vi "Init ST5520.vi"(8 "error in (no error)":errorcluster caption="entrée d'erreur (pas d'erreur)") -> (0 "error out":errorcluster caption="sortie d'erreur", 3 "Cluster Paramètres fichier Ini":T1)   [LabVIEW 2020]
uses:
  <vilib>/Utility/config.llb/Read Key (U32).vi
  <vilib>/Utility/config.llb/Read Key (String).vi
  <vilib>/Utility/config.llb/Read Key (Double).vi
  <vilib>/Utility/config.llb/NI_LVConfig.lvlib
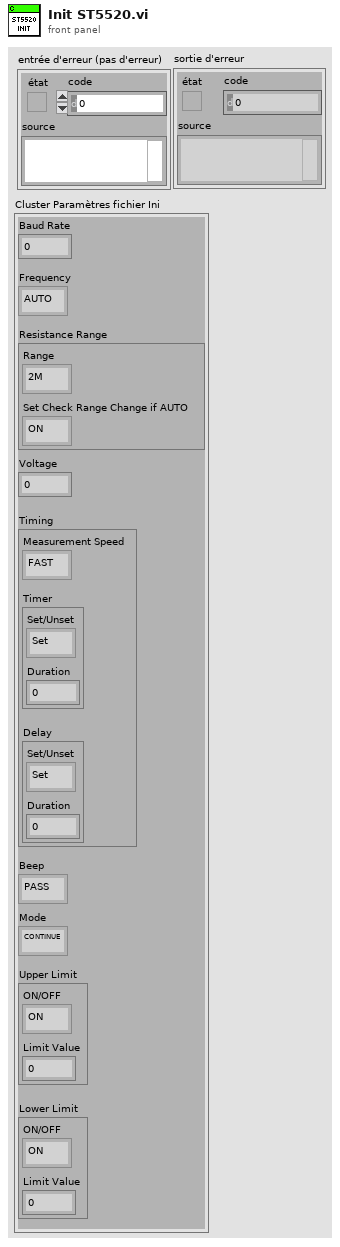
[diagram p1: front panel]
types:
  T1 = cluster{"Baud Rate":u32, "Frequency":enum8{"AUTO", "50", "60"}, "Resistance Range":cluster{"Range":enum16{"2M", "20M", "200M", "2000M", "4000M", "AUTO"}, "Set Check Range Change if AUTO":enum16{"ON", "OFF"}}, "Voltage":u16, "Timing":cluster{"Measurement Speed":enum16{"FAST", "SLOW"}, "Timer":cluster{"Set/Unset":enum8{"Set", "Unset"}, "Duration":dbl}, "Delay":cluster{"Set/Unset":enum8{"Set", "Unset"}, "Duration":dbl}}, "Beep":enum8{"PASS", "FAIL", "OFF", "END"}, "Mode":enum8{"CONTINUE", "PASSSTOP", "FAILSTOP", "SEQUENCE"}, "Upper Limit":cluster{"ON/OFF":enum8{"ON", "OFF"}, "Limit Value":dbl}, "Lower Limit":cluster{"ON/OFF":enum8{"ON", "OFF"}, "Limit Value":dbl}}
  T2 = cluster{"ON/OFF":enum8{"ON", "OFF"}, "Limit Value":dbl}
  T3 = cluster{"Measurement Speed":enum16{"FAST", "SLOW"}, "Timer":cluster{"Set/Unset":enum8{"Set", "Unset"}, "Duration":dbl}, "Delay":cluster{"Set/Unset":enum8{"Set", "Unset"}, "Duration":dbl}}
  T4 = cluster{"Set/Unset":enum8{"Set", "Unset"}, "Duration":dbl}
  T5 = cluster{"Range":enum16{"2M", "20M", "200M", "2000M", "4000M", "AUTO"}, "Set Check Range Change if AUTO":enum16{"ON", "OFF"}}
  T6 = enum8{"CONTINUE", "PASSSTOP", "FAILSTOP", "SEQUENCE"}
  T7 = enum16{"2M", "20M", "200M", "2000M", "4000M", "AUTO"}
  T8 = typedef "NI_LVConfig.lvlib/Config Data RefNum.ctl" = refnum<k1>
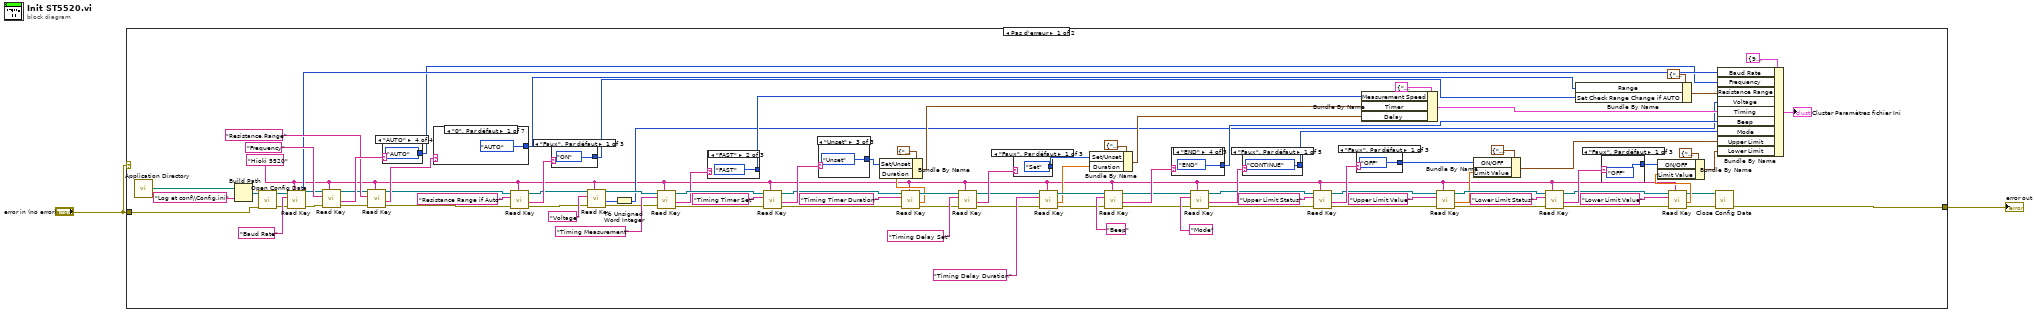
[diagram p0: block diagram]
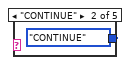
[diagram p2: hidden frame]
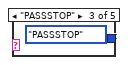
[diagram p3: hidden frame]
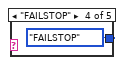
[diagram p4: hidden frame]
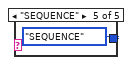
[diagram p5: hidden frame]
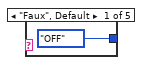
[diagram p6: hidden frame]
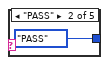
[diagram p7: hidden frame]
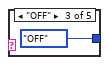
[diagram p8: hidden frame]
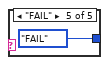
[diagram p9: hidden frame]
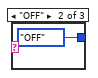
[diagram p10: hidden frame]
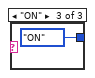
[diagram p11: hidden frame]
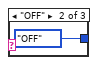
[diagram p12: hidden frame]
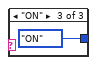
[diagram p13: hidden frame]
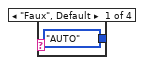
[diagram p14: hidden frame]
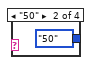
[diagram p15: hidden frame]
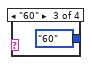
[diagram p16: hidden frame]
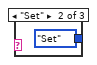
[diagram p17: hidden frame]
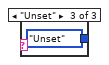
[diagram p18: hidden frame]
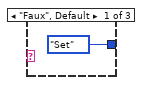
[diagram p19: hidden frame]
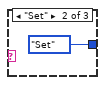
[diagram p20: hidden frame]
diagram:
  n1 = case shown="Pas d'erreur" "error in (no error)" {
    tunnel: "error in (no error)" -> [w5 w139]
    tunnel: [w4 w139] -> w2
    frame No Error {
      w7 = "Hioki 5520" ("section")
      n2 = call <vilib>:"Application Directory.vi"() -> ("Application Directory"=w3:path)
      n3 = Build Path(base path=w3, name or relative path="Log et conf\\Config.ini") -> (appended path=w43:path)
      n4 = call <vilib>:"Open Config Data.vi"("error in (no error)"=w5, "configuration file path"=w43) -> ("error out"=w6:errorcluster, "refnum"=w45:T8)  [unwired: 7 in, 1 out]
      n5 = call-poly <vilib>:"Read Key.vi"("section"=w7, "error in (no error)"=w6, "key"="Baud Rate", "refnum"=w45) -> ("error out"=w16:errorcluster, "value"=w41:u32, "refnum out"=w47:T8)  [unwired: 4 in, 1 out]
      n6 = call-poly <vilib>:"Read Key.vi"("section"=w7, "error in (no error)"=w16, "key"="Frequency", "refnum"=w47) -> ("error out"=w15:errorcluster, "value"=w68:string, "refnum out"=w48:T8)  [unwired: 4 in, 1 out]
      n7 = call-poly <vilib>:"Read Key.vi"("section"=w7, "error in (no error)"=w15, "key"="Resistance Range", "refnum"=w48) -> ("error out"=w14:errorcluster, "value"=w64:string, "refnum out"=w49:T8)  [unwired: 4 in, 1 out]
      n8 = case shown="\"AUTO\"" w68 {
        tunnel: [enum8{"AUTO", "50", "60"}."AUTO" ("Frequency") enum8{"AUTO", "50", "60"}."50" ("Frequency") enum8{"AUTO", "50", "60"}."60" ("Frequency") enum8{"AUTO", "50", "60"}."AUTO" ("Frequency")] -> w40
        frame "Faux", Default {
        }
        frame "50" {
        }
        frame "60" {
        }
        frame "AUTO" {
        }
      }
      n9 = case shown="\"0\", Par défaut" w64 {
        tunnel: [T7."AUTO" ("Range") T7."2M" ("Range") T7."20M" ("Range") T7."200M" ("Range") T7."2000M" ("Range") T7."4000M" ("Range") T7."AUTO" ("Range")] -> w39
        frame "0", Default {
        }
        frame "2M" {
        }
        frame "20M" {
        }
        frame "200M" {
        }
        frame "2000M" {
        }
        frame "4000M" {
        }
        frame "AUTO" {
        }
      }
      n10 = call-poly <vilib>:"Read Key.vi"("section"=w7, "error in (no error)"=w14, "key"="Resistance Range if Auto", "refnum"=w49) -> ("error out"=w13:errorcluster, "value"=w65:string, "refnum out"=w50:T8)  [unwired: 4 in, 1 out]
      n11 = case shown="\"Faux\", Par défaut" w65 {
        tunnel: [enum16{"ON", "OFF"}."ON" ("Set Check Range Change if AUTO") enum16{"ON", "OFF"}."ON" ("Set Check Range Change if AUTO") enum16{"ON", "OFF"}."OFF" ("Set Check Range Change if AUTO")] -> w38
        frame "Faux", Default {
        }
        frame "ON" {
        }
        frame "OFF" {
        }
      }
      n12 = call-poly <vilib>:"Read Key.vi"("section"=w7, "error in (no error)"=w13, "key"="Voltage", "refnum"=w50) -> ("error out"=w12:errorcluster, "value"=w27:u32, "refnum out"=w51:T8)  [unwired: 4 in, 1 out]
      n13 = To Unsigned Word Integer(number=w27) -> (unsigned 16bit integer=w26:u16)
      n14 = call-poly <vilib>:"Read Key.vi"("section"=w7, "error in (no error)"=w12, "key"="Timing Measurement", "refnum"=w51) -> ("error out"=w11:errorcluster, "value"=w46:string, "refnum out"=w52:T8)  [unwired: 4 in, 1 out]
      n15 = case shown="\"FAST\"" w46 {
        tunnel: [enum16{"FAST", "SLOW"}."SLOW" ("Measurement Speed") enum16{"FAST", "SLOW"}."FAST" ("Measurement Speed") enum16{"FAST", "SLOW"}."SLOW" ("Measurement Speed")] -> w37
        frame "Faux", Default {
        }
        frame "FAST" {
        }
        frame "SLOW" {
        }
      }
      n16 = call-poly <vilib>:"Read Key.vi"("section"=w7, "error in (no error)"=w11, "key"="Timing Timer Set", "refnum"=w52) -> ("error out"=w10:errorcluster, "value"=w66:string, "refnum out"=w53:T8)  [unwired: 4 in, 1 out]
      n17 = case shown="\"Unset\"" w66 {
        tunnel: [enum8{"Set", "Unset"}."Set" ("Set/Unset") enum8{"Set", "Unset"}."Set" ("Set/Unset") enum8{"Set", "Unset"}."Unset" ("Set/Unset")] -> w36
        frame "Faux", Default {
        }
        frame "Set" {
        }
        frame "Unset" {
        }
      }
      n18 = call-poly <vilib>:"Read Key.vi"("section"=w7, "error in (no error)"=w10, "key"="Timing Timer Duration", "refnum"=w53) -> ("error out"=w9:errorcluster, "value"=w30:dbl, "refnum out"=w63:T8)  [unwired: 4 in, 1 out]
      n19 = Bundle By Name(cluster=T4 {"Set/Unset"=enum."Set", "Duration"=60.0} ("Timer"), "Set/Unset"=w36, "Duration"=w30) -> (w90:T4)
      n20 = call-poly <vilib>:"Read Key.vi"("section"=w7, "error in (no error)"=w9, "key"="Timing Delay Set", "refnum"=w63) -> ("error out"=w8:errorcluster, "value"=w67:string, "refnum out"=w54:T8)  [unwired: 4 in, 1 out]
      n21 = case shown="\"Faux\", Par défaut" w67 {
        tunnel: [enum8{"Set", "Unset"}."Set" ("Set/Unset") enum8{"Set", "Unset"}."Set" ("Set/Unset") enum8{"Set", "Unset"}."Unset" ("Set/Unset")] -> w86
        frame "Faux", Default {
        }
        frame "Set" {
        }
        frame "Unset" {
        }
      }
      n22 = call-poly <vilib>:"Read Key.vi"("section"=w7, "error in (no error)"=w8, "key"="Timing Delay Duration", "refnum"=w54) -> ("error out"=w17:errorcluster, "value"=w29:dbl, "refnum out"=w69:T8)  [unwired: 4 in, 1 out]
      n23 = Bundle By Name(cluster=T4 {"Set/Unset"=enum."Set", "Duration"=0.0} ("Delay"), "Set/Unset"=w86, "Duration"=w29) -> (w91:T4)
      n24 = call-poly <vilib>:"Read Key.vi"("section"=w7, "error in (no error)"=w17, "key"="Beep", "refnum"=w69) -> ("error out"=w18:errorcluster, "value"=w83:string, "refnum out"=w76:T8)  [unwired: 4 in, 1 out]
      n25 = case shown="\"END\"" w83 {
        tunnel: [enum8{"PASS", "FAIL", "OFF", "END"}."OFF" ("Beep") enum8{"PASS", "FAIL", "OFF", "END"}."PASS" ("Beep") enum8{"PASS", "FAIL", "OFF", "END"}."OFF" ("Beep") enum8{"PASS", "FAIL", "OFF", "END"}."END" ("Beep") enum8{"PASS", "FAIL", "OFF", "END"}."FAIL" ("Beep")] -> w28
        frame "Faux", Default {
        }
        frame "PASS" {
        }
        frame "OFF" {
        }
        frame "END" {
        }
        frame "FAIL" {
        }
      }
      n26 = call-poly <vilib>:"Read Key.vi"("section"=w7, "error in (no error)"=w18, "key"="Mode", "refnum"=w76) -> ("error out"=w19:errorcluster, "value"=w84:string, "refnum out"=w77:T8)  [unwired: 4 in, 1 out]
      n27 = case shown="\"Faux\", Par défaut" w84 {
        tunnel: [T6."CONTINUE" ("Mode") T6."CONTINUE" ("Mode") T6."PASSSTOP" ("Mode") T6."FAILSTOP" ("Mode") T6."SEQUENCE" ("Mode")] -> w31
        frame "Faux", Default {
        }
        frame "CONTINUE" {
        }
        frame "PASSSTOP" {
        }
        frame "FAILSTOP" {
        }
        frame "SEQUENCE" {
        }
      }
      n28 = call-poly <vilib>:"Read Key.vi"("section"=w7, "error in (no error)"=w19, "key"="Upper Limit Status", "refnum"=w77) -> ("error out"=w20:errorcluster, "value"=w81:string, "refnum out"=w78:T8)  [unwired: 4 in, 1 out]
      n29 = case shown="\"Faux\", Par défaut" w81 {
        tunnel: [enum8{"ON", "OFF"}."OFF" ("ON/OFF") enum8{"ON", "OFF"}."OFF" ("ON/OFF") enum8{"ON", "OFF"}."ON" ("ON/OFF")] -> w32
        frame "Faux", Default {
        }
        frame "OFF" {
        }
        frame "ON" {
        }
      }
      n30 = Bundle By Name(cluster=T3 {"Measurement Speed"=enum."FAST", "Timer"={"Set/Unset"=enum."Set", "Duration"=0.045}, "Delay"={"Set/Unset"=enum."Set", "Duration"=0.045}} ("Timing"), "Measurement Speed"=w37, "Timer"=w90, "Delay"=w91) -> (w96:T3)
      n31 = call-poly <vilib>:"Read Key.vi"("section"=w7, "error in (no error)"=w20, "key"="Upper Limit Value", "refnum"=w78) -> ("error out"=w21:errorcluster, "value"=w33:dbl, "refnum out"=w79:T8)  [unwired: 4 in, 1 out]
      n32 = Bundle By Name(cluster=T2 {"ON/OFF"=enum."ON", "Limit Value"=0.045} ("cluster d'entrée"), "ON/OFF"=w32, "Limit Value"=w33) -> (w97:T2)
      n33 = call-poly <vilib>:"Read Key.vi"("section"=w7, "error in (no error)"=w21, "key"="Lower Limit Status", "refnum"=w79) -> ("error out"=w22:errorcluster, "value"=w82:string, "refnum out"=w80:T8)  [unwired: 4 in, 1 out]
      n34 = Bundle By Name(cluster=T5 {"Range"=enum."2M", "Set Check Range Change if AUTO"=enum."ON"} ("Resistance Range"), "Range"=w39, "Set Check Range Change if AUTO"=w38) -> (w95:T5)
      n35 = case shown="\"Faux\", Par défaut" w82 {
        tunnel: [enum8{"ON", "OFF"}."OFF" ("ON/OFF") enum8{"ON", "OFF"}."OFF" ("ON/OFF") enum8{"ON", "OFF"}."ON" ("ON/OFF")] -> w34
        frame "Faux", Default {
        }
        frame "OFF" {
        }
        frame "ON" {
        }
      }
      n36 = call-poly <vilib>:"Read Key.vi"("section"=w7, "error in (no error)"=w22, "key"="Lower Limit Value", "refnum"=w80) -> ("error out"=w23:errorcluster, "value"=w35:dbl, "refnum out"=w25:T8)  [unwired: 4 in, 1 out]
      n37 = Bundle By Name(cluster=T2 {"ON/OFF"=enum."ON", "Limit Value"=0.045} ("cluster d'entrée"), "ON/OFF"=w34, "Limit Value"=w35) -> (w98:T2)
      n38 = call <vilib>:"Close Config Data.vi"("error in (no error)"=w23, "refnum"=w25) -> ("error out"=w4:errorcluster)  [unwired: 8 in, 1 out]
      n39 = Bundle By Name(cluster=T1 {"Baud Rate"=9600, "Frequency"=enum."AUTO", "Resistance Range"={"Range"=enum."2M", "Set Check Range Change if AUTO"=enum."ON"}, "Voltage"=25, "Timing"={"Measurement Speed"=enum."FAST", "Timer"={"Set/Unset"=enum."Set", "Duration"=0.045}, "Delay"={"Set/Unset"=enum."Set", "Duration"=0.045}}, "Beep"=enum."PASS", "Mode"=enum."CONTINUE", "Upper Limit"={"ON/OFF"=enum."ON", "Limit Value"=0.045}, "Lower Limit"={"ON/OFF"=enum."ON", "Limit Value"=0.045}}, "Baud Rate"=w41, "Frequency"=w40, "Resistance Range"=w95, "Voltage"=w26, "Timing"=w96, "Beep"=w28, "Mode"=w31, "Upper Limit"=w97, "Lower Limit"=w98) -> (→"Cluster Paramètres fichier Ini":T1)
    }
    frame Error {
    }
  }
  "error out" <- w2
